vi "Stop.vi"(8 "error in (no error)":errorcluster, 11 "NEO480HTA Base CFG in":refnum<class "Read All CFG.lvclass">) -> (0 "error out":errorcluster, 3 "NEO480HTA Base CFG out":refnum<class "Read All CFG.lvclass">)   [LabVIEW 2023]
uses:
  Read All CFG.lvclass
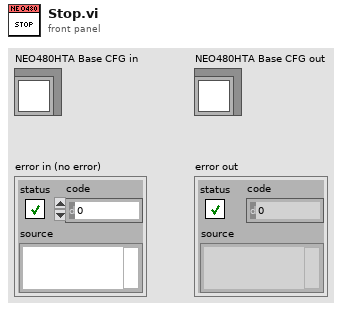
[diagram p1: front panel]
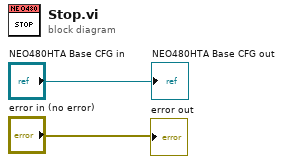
[diagram p0: block diagram]
diagram:
  "error out" <- "error in (no error)"
  "NEO480HTA Base CFG out" <- "NEO480HTA Base CFG in"
